vi "Untitled 1.vi"() -> ()   [LabVIEW 2018]
panel:
  in  "Image Rotation:":enum16{"0", "90", "180", "-90"}(ring)
  out "Serial":string
  in  "serial?":bool
  in  "Color":bool
  in  "Live":bool
  in  "stop":bool
  out "Devices":string[](array[string])
  in  "ICImagingControl":refnum<k7>(container)
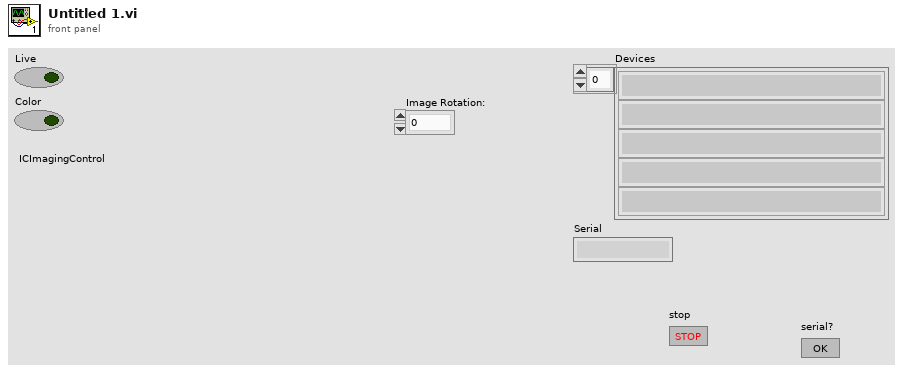
[diagram p1: front panel]
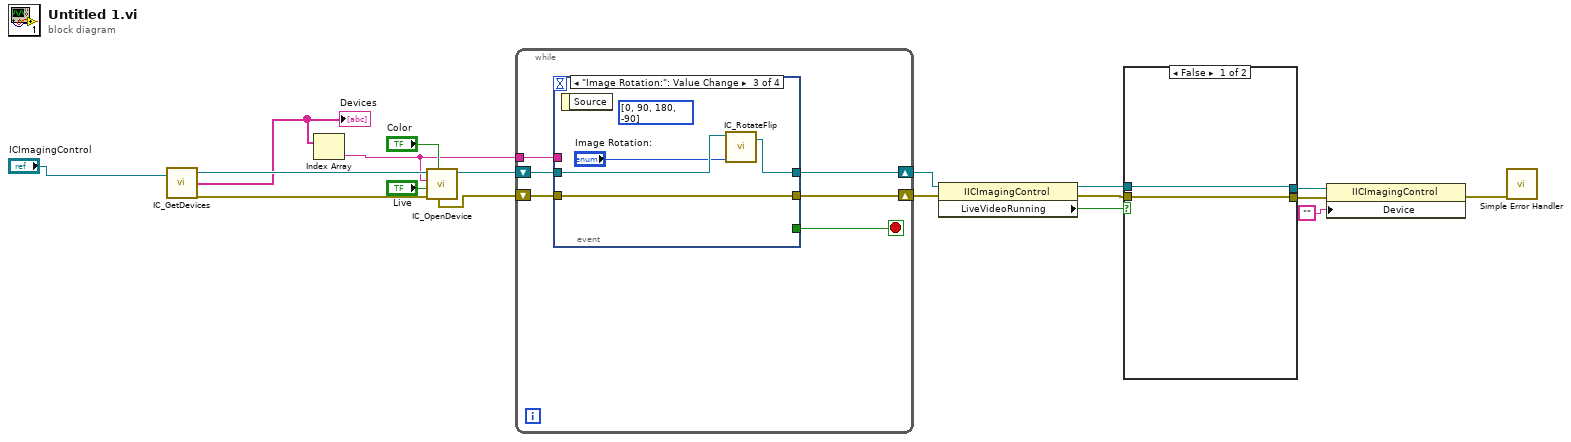
[diagram p0: block diagram]
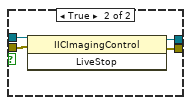
[diagram p2: hidden frame]
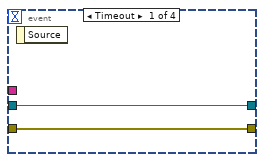
[diagram p3: hidden frame]
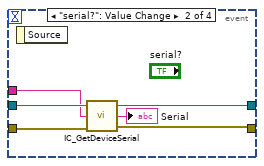
[diagram p4: hidden frame]
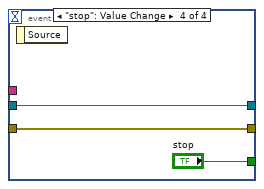
[diagram p5: hidden frame]
diagram:
  n1 = call <userlib>:"IC_GetDevices.vi"("ICImagingControl In"="ICImagingControl") -> ("ICImagingControl Out"=w18:refnum<k7>, "Devices"=w4:string[], "Error Out"=w17:errorcluster)  [unwired: 1 in]
  "Devices" <- w4
  n2 = Index Array(array=w4) -> (element=w3:string)  [unwired: 1 in]
  n3 = call <userlib>:"IC_OpenDevice.vi"("Color"="Color", "Error In (no error)"=w17, "Live"="Live", "Device"=w3, "ICImagingControl In"=w18) -> ("ICImagingControl Out"=w16:refnum<k7>, "Error Out"=w15:errorcluster)  [unwired: 1 in, 4 out]
  n4 = while {
    shift-right: [w23] -> w11
    shift-left: w15 -> [w24]
    shift-right: [w20] -> w12
    shift-left: w16 -> [w22]
    tunnel: w3 -> [w19]
    stop <- w21 stop-if-true
    n5 = event shown="[2] \"Image Rotation:\": Value Change" {
      selector: _ -> [_ _ _ _]
      dyn-events: _ -> [_ _ _ _]
      timeout: _ -> [_ _ _ _]
      tunnel: w24 -> [w26 w31 w36 w39]
      tunnel: [w26 w28 w36 w39] -> w23
      tunnel: w22 -> [w25 w32 w35 w37]
      tunnel: [_ _ _ "stop"] -> w21
      tunnel: [w25 w29 w34 w37] -> w20
      tunnel: w19 -> [_ w30 _ _]
      event Timeout {
        n6 = event-data() -> ()  [unwired: 1 in, 1 out]
      }
      event "serial?": Value Change {
        n7 = event-data() -> ()  [unwired: 1 in, 1 out]
        n8 = call <userlib>:"IC_GetDeviceSerial.vi"("Error In (no error)"=w31, "Device"=w30, "ICImagingControl In"=w32) -> ("Error Out"=w28:errorcluster, "Serial"=→"Serial":string, "ICImagingControl Out"=w29:refnum<k7>)
      }
      event "Image Rotation:": Value Change {
        (unwired) i16[] [0, 90, 180, -90]
        n9 = event-data() -> ()  [unwired: 1 in, 1 out]
        n10 = call <userlib>:"IC_RotateFlip.vi"("Rotation angle"="Image Rotation:", "ICImagingControl"=w35) -> ("ICImagingControl 3"=w34:refnum<k7>)  [unwired: 2 in, 1 out]
      }
      event "stop": Value Change {
        n11 = event-data() -> ()  [unwired: 1 in, 1 out]
      }
    }
  }
  n12 = property class="IICImagingControl"(reference=w12, error in=w11) -> (reference out=w9:refnum<k7>, error out=w8:errorcluster, "LiveVideoRunning"=w10:bool)
  n13 = case shown="False" w10 {
    tunnel: w9 -> [w41 w45]
    tunnel: w8 -> [w40 w44]
    tunnel: [w40 w43] -> w7
    tunnel: [w41 w42] -> w6
    frame False {
    }
    frame True {
      n14 = invoke class="IICImagingControl" method="LiveStop"(reference=w45, error in=w44) -> (reference out=w42:refnum<k7>, error out=w43:errorcluster)  [unwired: 1 in, 1 out]
    }
  }
  n15 = property class="IICImagingControl"(reference=w6, error in=w7, "Device"="") -> (error out=w1:errorcluster)  [unwired: 1 out]
  n16 = call <vilib>:"Simple Error Handler.vi"("error in (no error)"=w1) -> ()  [unwired: 4 in, 5 out]
